vi "Check Log File.vi"(8 "Error In":errorcluster, 11 "Log File Path":path) -> (0 "Error Out":errorcluster)   [LabVIEW 2015]
doc: "Check if log file Exist. If not, it will be created."
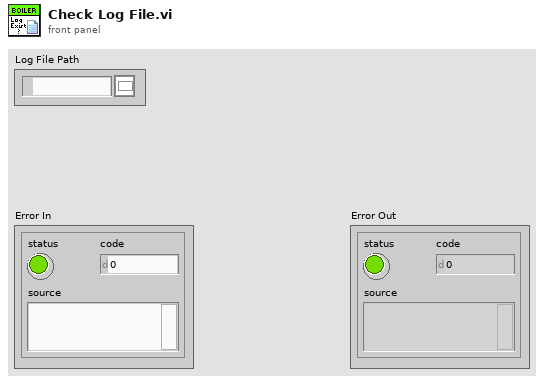
[diagram p1: front panel]
types:
  T1 = enum16{"open", "replace", "create", "open or create", "replace or create", "replace or create with confirmation"}
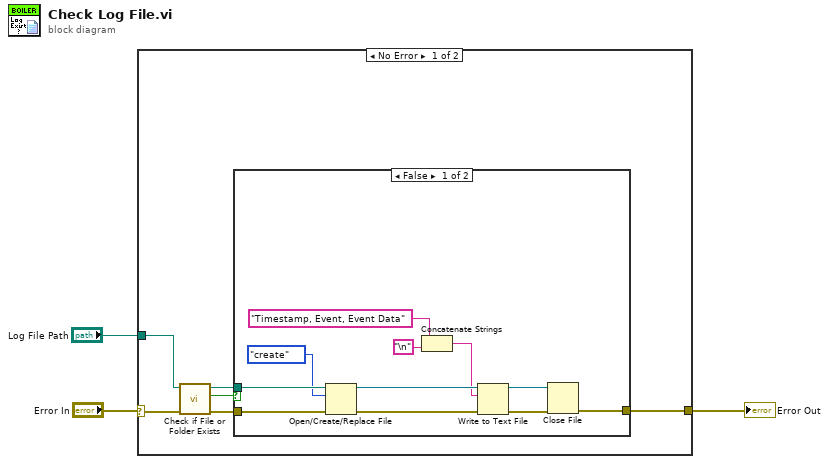
[diagram p0: block diagram]
diagram:
  n1 = case shown="No Error" "Error In" {
    selector: "Error In" -> [w9 w22]
    tunnel: "Log File Path" -> [w8 _]
    tunnel: [w4 w22] -> w1
    frame No Error {
      n2 = call <vilib>:"Check if File or Folder Exists.vi"("error in (no error)"=w9, "path"=w8) -> ("error out"=w5:errorcluster, "file or folder exists?"=w7:bool, "dup path"=w6:path)  [unwired: 7 in]
      n3 = case shown="False" w7 {
        tunnel: w6 -> [w20 _]
        tunnel: w5 -> [w18 w21]
        tunnel: [w13 w21] -> w4
        frame False {
          n4 = Open/Create/Replace File(file path (use dialog)=w20, error in=w18, operation (0:open)=T1."create") -> (refnum out=w16:refnum<file>, error out=w17:errorcluster)  [unwired: 3 in, 1 out]
          n5 = Concatenate Strings("Timestamp, Event, Event Data" ("text"), "\n") -> (w10:string)
          n6 = Write to Text File(file (use dialog)=w16, text=w10, error in=w17) -> (refnum out=w14:refnum<file>, error out=w15:errorcluster)  [unwired: 1 in, 1 out]
          n7 = Close File(refnum=w14, error in=w15) -> (error out=w13:errorcluster)  [unwired: 1 out]
        }
        frame True {
        }
      }
    }
    frame Error {
    }
  }
  "Error Out" <- w1
